vi "MMEM_DAT.vi"(0 "VISA IN":refnum<visa-resource-name>, 1 "FilePath":string, 5 "error in":errorcluster, 9 "HrsToFlag":dbl=24.0) -> (8 "=>SelectedHrs?(t)":bool, 12 "File Date/Time":string, 14 "VISA Out":refnum<visa-resource-name>, 19 "error out":errorcluster)   [LabVIEW 2018]
doc: "MMEMory:CATalog[:<char>]? [<folder>] \n1608\n\n(Read-only) Returns a comma-separated string of file names that are in the specified folder. If there \nare no files of the specified type, \"NO CATALOG\" is returned. Learn about File Types \nParameters \n<char> The type of files to list. Choose from: \nSTATe - Instrument states (.sta) \nCORRection - Calibration Data (.cal) \nCSARchive - Instrument state and calibration data (.csa) \nCSTate - Instrument state and link to Calibration data (.cst) \nIf unspecified then ALL file types (even unknown types) are listed. \n<folder> String - Any existing folder name. See Specifying Path Names \nExamples MMEM:CAT? 'lists all files from the current folder \nmmemory:catalog:correction? 'C:\\Program Files\\Agilent\\Network \nAnalyzer\\Documents' 'lists .cal files from the specified folder \nDefault Not applicable"
panel:
  out "x-y":dbl
  out "output 2":dbl
  out "File Date/Time":timestamp
  out "Date":string
  out "d":string
  out "m":string
  out "Y":string
  out "array":string[](array[string])
  out "output 1":dbl
  out "Time":string
  # "This vi will check the age of a file and throw a flag if the file is older than HRS specified"
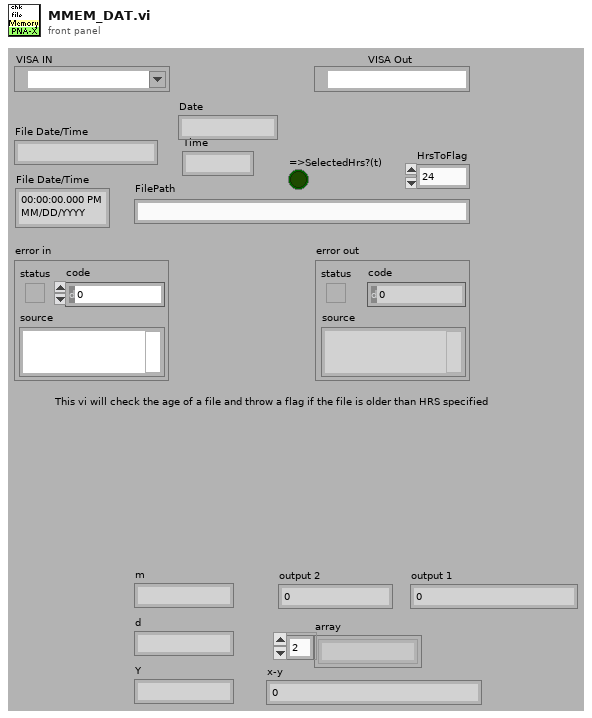
[diagram p1: front panel]
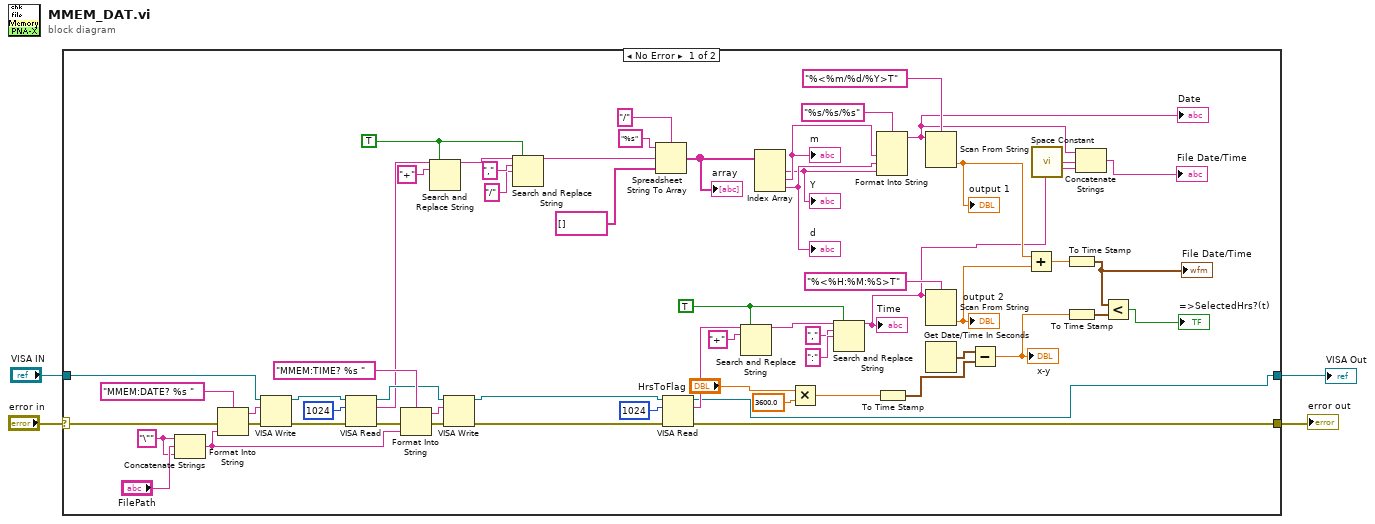
[diagram p0: block diagram]
diagram:
  n1 = case shown="No Error" "error in" {
    selector: "error in" -> [w64 w66]
    tunnel: [w5 w66] -> w1
    tunnel: [w6 w65] -> w2
    tunnel: "VISA IN" -> [w47 w65]
    frame No Error {
      w39 = TRUE ("replace all? (F)")
      w40 = TRUE ("replace all? (F)")
      w56 = "\"" ("string")
      n2 = Concatenate Strings(w56, "FilePath", w56) -> (w49:string)
      n3 = Format Into String(format string="MMEM:DATE? %s " ("Cmdline"), error in=w64, w49) -> (resulting string=w62:string, error out=w63:errorcluster)  [unwired: 1 in]
      n4 = VISA Write(VISA resource name=w47, write buffer=w62, error in (no error)=w63) -> (VISA resource name out=w58:refnum<visa-resource-name>, error out=w60:errorcluster)  [unwired: 1 out]
      n5 = VISA Read(VISA resource name=w58, byte count=1024, error in (no error)=w60) -> (VISA resource name out=w48:refnum<visa-resource-name>, read buffer=w45:string, error out=w46:errorcluster)  [unwired: 1 out]
      n6 = Format Into String(format string="MMEM:TIME? %s " ("Cmdline"), error in=w46, w49) -> (resulting string=w51:string, error out=w50:errorcluster)  [unwired: 1 in]
      n7 = Search and Replace String(replace all?=w40, input string=w45, search string="+") -> (result string=w43:string)  [unwired: 5 in, 3 out]
      n8 = VISA Write(VISA resource name=w48, write buffer=w51, error in (no error)=w50) -> (VISA resource name out=w55:refnum<visa-resource-name>, error out=w53:errorcluster)  [unwired: 1 out]
      n9 = Search and Replace String(replace all?=w40, input string=w43, search string=",", replace string="/" ("search string")) -> (result string=w32:string)  [unwired: 4 in, 3 out]
      n10 = Spreadsheet String To Array(delimiter (Tab)="/", format string="%s", spreadsheet string=w32, array type (2D Dbl)=string[] []) -> (array=w28:string[])
      "array" <- w28
      n11 = VISA Read(VISA resource name=w55, byte count=1024, error in (no error)=w53) -> (VISA resource name out=w6:refnum<visa-resource-name>, read buffer=w34:string, error out=w5:errorcluster)  [unwired: 1 out]
      n12 = Search and Replace String(replace all?=w39, input string=w34, search string="+") -> (result string=w36:string)  [unwired: 5 in, 3 out]
      n13 = Index Array(array=w28) -> (element #1=w25:string, element #2=w27:string, element #3=w26:string)  [unwired: 3 in]
      "Y" <- w25
      "m" <- w27
      "d" <- w26
      n14 = Multiply(x="HrsToFlag", y=3600.0) -> (x*y=w15:dbl)
      n15 = Search and Replace String(replace all?=w39, input string=w36, search string=",", replace string=":" ("search string")) -> (result string=w12:string)  [unwired: 4 in, 3 out]
      "Time" <- w12
      n16 = Format Into String(format string="%s/%s/%s", w27, w26, w25) -> (resulting string=w9:string)  [unwired: 2 in, 1 out]
      "Date" <- w9
      n17 = To Time Stamp(1:w15) -> (0:w19:timestamp)
      n18 = Scan From String(format string="%<%m/%d/%Y>T", input string=w9) -> (output 1=w22:dbl)  [unwired: 3 in, 3 out]
      "output 1" <- w22
      n19 = Scan From String(format string="%<%H:%M:%S>T", input string=w12) -> (output 1=w21:dbl)  [unwired: 3 in, 3 out]
      "output 2" <- w21
      n20 = Get Date/Time In Seconds() -> (seconds since 1Jan1904=w18:timestamp)
      n21 = Subtract(x=w18, y=w19) -> (x-y=w17:dbl)
      "x-y" <- w17
      n22 = Add(x=w22, y=w21) -> (x+y=w20:dbl)
      n23 = call <vilib>:"Space Constant.vi"() -> ("String"=w11:string)
      n24 = To Time Stamp(1:w20) -> (0:w10:timestamp)
      "File Date/Time" <- w10
      n25 = To Time Stamp(1:w17) -> (0:w16:timestamp)
      n26 = Concatenate Strings(w9, w11, w12) -> (→"File Date/Time":string)
      n27 = Less?(x=w10, y=w16) -> (x < y?=→"=>SelectedHrs?(t)":bool)
    }
    frame Error {
    }
  }
  "VISA Out" <- w2
  "error out" <- w1
